vi "Create.vi"(8 "error in (no error)":errorcluster, 11 "bitfile":path) -> (0 "error out":errorcluster, 1 "bitfile major version":T1, 2 "IPs":refnum<class "Engine Simulation IP.lvclass">[](array[class]), 3 "Engine Simulation Session out":refnum<class "Engine Simulation Session.lvclass">, 5 "bitfile full version":string)   [LabVIEW 2013, in "Engine Simulation Session.lvclass"]
uses:
  Engine Simulation Session.lvclass
  Engine Simulation IP.lvclass
  Bitfile Major Version.ctl
  session class private data.ctl
  Engine Simulation Session.lvclass/Engine Simulation Session.ctl
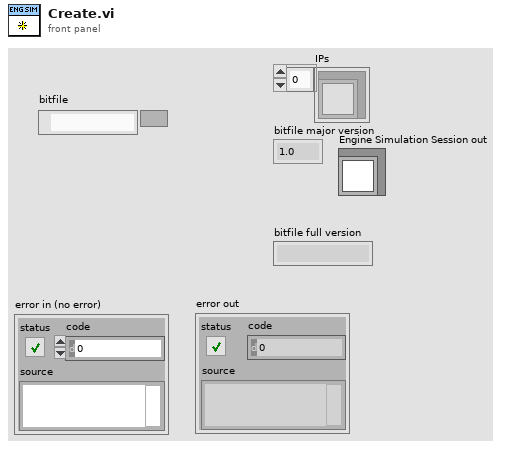
[diagram p1: front panel]
types:
  T1 = typedef "Engine Simulation Session.lvclass/Bitfile Major Version.ctl" = enum16{"1.0", "1.1", "1.2", "1.3"}
  T2 = typedef "Engine Simulation Session.lvclass/session class private data.ctl" = cluster{"running":bool, "fpga reference":refnum<k20>, "bitfile":path}
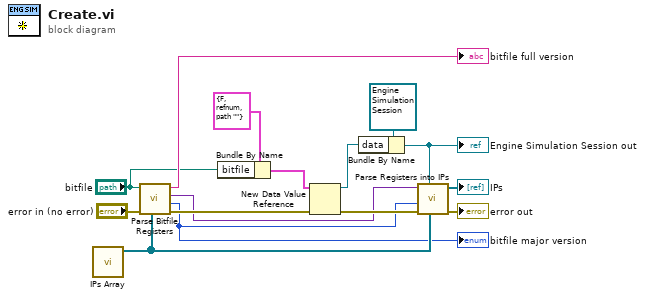
[diagram p0: block diagram]
diagram:
  n1 = call "IPs Array.vi"() -> ("IPs"=w6:refnum<class "Engine Simulation IP.lvclass">[])  [unwired: 11 in]
  n2 = call "Parse Bitfile Registers.vi"("IP Classes"=w6, "error in (no error)"="error in (no error)", "bitfile"="bitfile") -> ("error out"=w11:errorcluster, "EST version"=w4:T1, "reg LUT"=w3:variant, "EST version string"=→"bitfile full version":string)  [unwired: 5 in]
  "bitfile major version" <- w4
  n3 = Bundle By Name(cluster=T2 {"running"=FALSE, "fpga reference"=refnum, "bitfile"=path ""} ("Cluster of class private data"), "bitfile"="bitfile") -> (w2:T2)
  n4 = New Data Value Reference(data value=w2, error in=w11) -> (data value reference=w12:refnum<data-value>, error out=w10:errorcluster)
  n5 = Bundle By Name(cluster=refnum<class "Engine Simulation Session.lvclass"> refnum ("Engine Simulation Session.lvclass"), "data"=w12) -> (w8:refnum<class "Engine Simulation Session.lvclass">)
  "Engine Simulation Session out" <- w8
  n6 = call "Parse Registers into IPs.vi"("IP Types"=w6, "engine simulation session in"=w8, "error in (no error)"=w10, "Version"=w4, "Registers LUT"=w3) -> ("error out"=→"error out":errorcluster, "IPs"=→"IPs":refnum<class "Engine Simulation IP.lvclass">[])  [unwired: 5 in]
